vi "Start Server.vi"(8 "error in (no error)":errorcluster, 11 "Server Fixture in":refnum<class "Server Fixture.lvclass">) -> (0 "error out":errorcluster, 3 "Server Fixture out":refnum<class "Server Fixture.lvclass">)   [LabVIEW 2013, in "libssh2_integration_tests.lvlib" / "Server Fixture.lvclass"]
uses:
  Server Fixture.lvclass
  Server Fixture.lvclass/Server Fixture.ctl
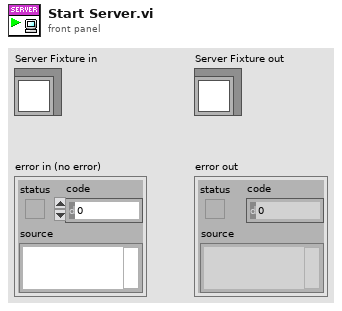
[diagram p1: front panel]
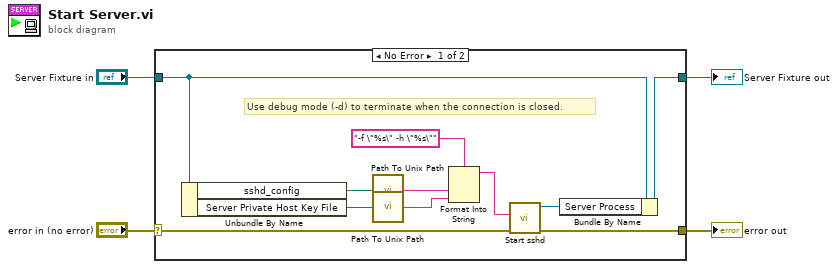
[diagram p0: block diagram]
diagram:
  n1 = case shown="No Error" "error in (no error)" {
    selector: "error in (no error)" -> [w6 w17]
    tunnel: [w5 w17] -> w3
    tunnel: [w7 w16] -> w1
    tunnel: "Server Fixture in" -> [w8 w16]
    frame No Error {
      # "Use debug mode (-d) to terminate when the connection is closed."
      n2 = Unbundle By Name(w8) -> ("sshd_config"=w11:path, "Server Private Host Key File"=w10:path)
      n3 = call "Path To Unix Path.vi"("path"=w11) -> ("unix path"=w13:string)  [unwired: 1 in]
      n4 = call "Path To Unix Path.vi"("path"=w10) -> ("unix path"=w14:string)  [unwired: 1 in]
      n5 = Format Into String(format string="-f \"%s\" -h \"%s\"" ("command line"), w13, w14) -> (resulting string=w12:string)  [unwired: 2 in, 1 out]
      n6 = call "Start sshd.vi"("error in (no error)"=w6, "arguments"=w12) -> ("error out"=w5:errorcluster, "Process"=w9:refnum<k24>)  [unwired: 8 in]
      n7 = Bundle By Name(cluster=w8, "Server Process"=w9) -> (w7:refnum<class "Server Fixture.lvclass">)
    }
    frame Error {
    }
  }
  "error out" <- w3
  "Server Fixture out" <- w1
